vi "InitFormatGlobals.vi"(8 "error in (no error)":errorcluster) -> (0 "error out":errorcluster)   [LabVIEW 2023]
doc: "Initializes the values of the Format globals."
uses:
  StringFormatGlobals.vi
panel:
  # "Initializes Format Globals"
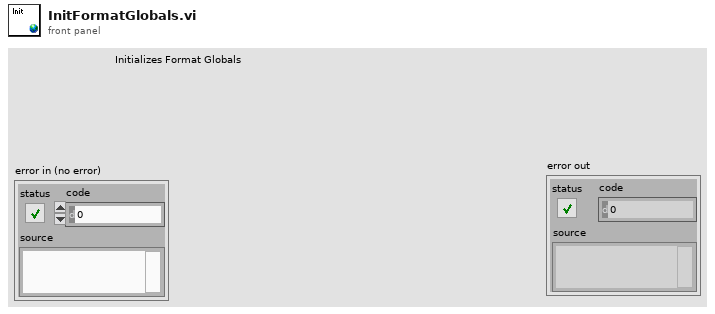
[diagram p1: front panel]
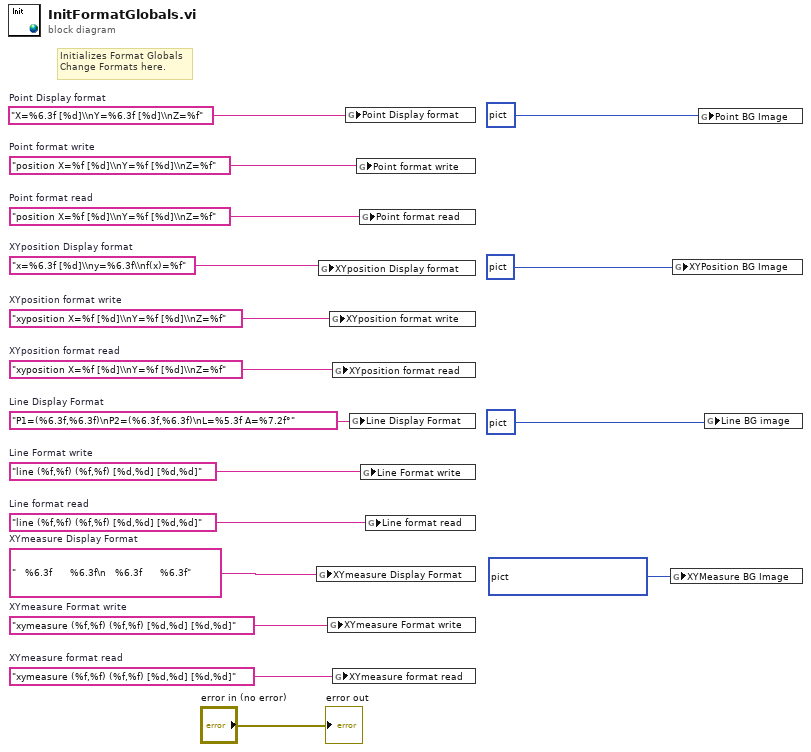
[diagram p0: block diagram]
diagram:
  w5 = "x=%6.3f [%d]\\ny=%6.3f\\nf(x)=%f"  # XYposition Display format
  w6 = "xyposition X=%f [%d]\\nY=%f [%d]\\nZ=%f"  # XYposition format read
  w7 = "xyposition X=%f [%d]\\nY=%f [%d]\\nZ=%f"  # XYposition format write
  w8 = "   %6.3f      %6.3f\n   %6.3f      %6.3f"  # XYmeasure Display Format
  w9 = "xymeasure (%f,%f) (%f,%f) [%d,%d] [%d,%d]"  # XYmeasure Format write
  w10 = "xymeasure (%f,%f) (%f,%f) [%d,%d] [%d,%d]"  # XYmeasure format read
  w12 = "position X=%f [%d]\\nY=%f [%d]\\nZ=%f"  # Point format write
  w13 = "position X=%f [%d]\\nY=%f [%d]\\nZ=%f"  # Point format read
  w14 = "X=%6.3f [%d]\\nY=%6.3f [%d]\\nZ=%f"  # Point Display format
  w15 = "line (%f,%f) (%f,%f) [%d,%d] [%d,%d]"  # Line format read
  w16 = "line (%f,%f) (%f,%f) [%d,%d] [%d,%d]"  # Line Format write
  w17 = "P1=(%6.3f,%6.3f)\nP2=(%6.3f,%6.3f)\nL=%5.3f A=%7.2f°"  # Line Display Format
  # "Initializes Format Globals\nChange Formats here."
  n1 = global write "StringFormatGlobals.vi" "XYmeasure Display Format"(w8) -> ()
  n2 = global write "StringFormatGlobals.vi" "XYposition Display format"(w5) -> ()
  n3 = global write "StringFormatGlobals.vi" "XYmeasure Format write"(w9) -> ()
  n4 = global write "StringFormatGlobals.vi" "XYposition format write"(w7) -> ()
  n5 = global write "StringFormatGlobals.vi" "XYposition format read"(w6) -> ()
  n6 = global write "StringFormatGlobals.vi" "XYmeasure format read"(w10) -> ()
  n7 = global write "StringFormatGlobals.vi" "Point Display format"(w14) -> ()
  n8 = global write "StringFormatGlobals.vi" "Line Display Format"(w17) -> ()
  n9 = global write "StringFormatGlobals.vi" "Point format write"(w12) -> ()
  n10 = global write "StringFormatGlobals.vi" "Point format read"(w13) -> ()
  n11 = global write "StringFormatGlobals.vi" "Line Format write"(w16) -> ()
  n12 = global write "StringFormatGlobals.vi" "Line format read"(w15) -> ()
  n13 = global write "StringFormatGlobals.vi" "XYMeasure BG Image"(picture bytes[220] ("new picture")) -> ()
  n14 = global write "StringFormatGlobals.vi" "XYPosition BG Image"(picture data[5B] ("XYPosition BG Image")) -> ()
  n15 = global write "StringFormatGlobals.vi" "Point BG Image"(picture data[5B] ("Point BG Image")) -> ()
  n16 = global write "StringFormatGlobals.vi" "Line BG image"(picture data[5B] ("Line BG image")) -> ()
  "error out" <- "error in (no error)"
